vi "simulando_tempratura.vi"() -> ()   [LabVIEW 2013]
panel:
  in  "Delay (sec)":dbl format="%#_13g"
  in  "Numero de Medições":i32
  out "Gradico de Temperatura":cluster{i32[], dbl[]}(graph)
  out "Termometro":dbl(slide) scale=0.0..100.0
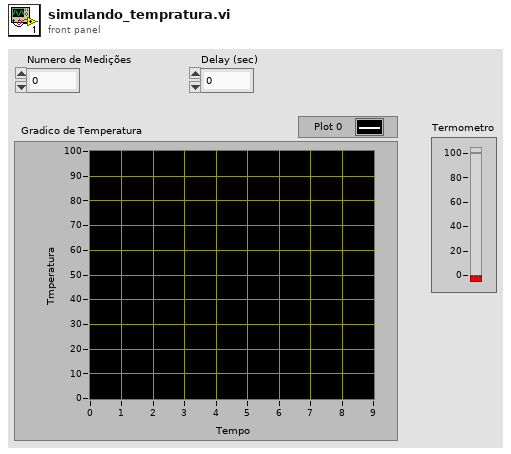
[diagram p1: front panel]
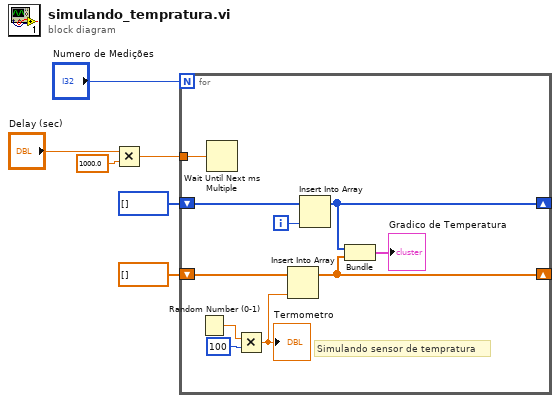
[diagram p0: block diagram]
diagram:
  n1 = Multiply(x="Delay (sec)", y=1000.0) -> (x*y=w3:dbl)
  n2 = for {
    N: "Numero de Medições" -> [_]
    tunnel: w3 -> [w16]
    shift-right: [w11] -> _
    shift-left: i32[] [] -> [w12]
    shift-right: [w8] -> _
    shift-left: dbl[] [] -> [w9]
    i -> [w13]
    # "Simulando sensor de tempratura"
    n3 = Random Number (0-1)() -> (number: 0 to 1=w15:dbl)
    n4 = Wait Until Next ms Multiple(millisecond multiple=w16) -> ()  [unwired: 1 out]
    n5 = Multiply(x=w15, y=100) -> (x*y=w10:dbl)
    "Termometro" <- w10
    n6 = Insert Into Array(array=w9, new element=w10) -> (w8:dbl[])  [unwired: 1 in]
    n7 = Insert Into Array(array=w12, new element=w13) -> (w11:i32[])  [unwired: 1 in]
    n8 = Bundle(w11, w8) -> (→"Gradico de Temperatura":cluster{i32[], dbl[]})  [unwired: 1 in]
  }
